vi "Convert_to_1D_Array.vi"(11 "Path":path) -> (3 "Array":string[](array[string]))   [LabVIEW 2017]
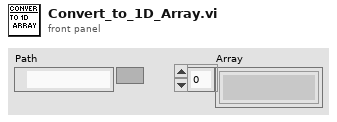
[diagram p1: front panel]
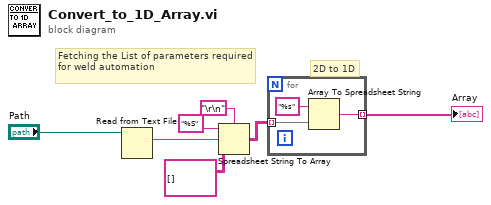
[diagram p0: block diagram]
diagram:
  # "2D to 1D"
  # "Fetching the List of parameters required for weld automation"
  n1 = Read from Text File(file (use dialog)="Path") -> (text=w2:string)  [unwired: 3 in, 3 out]
  n2 = Spreadsheet String To Array(delimiter (Tab)="\r\n", format string="%S", spreadsheet string=w2, array type (2D Dbl)=string[][] []) -> (array=w5:string[][])
  n3 = for {
    tunnel: w5 -> [w10] mode=indexing
    tunnel: [w8] -> w6 mode=indexing
    n4 = Array To Spreadsheet String(array=w10, 3:"%s" ("format string")) -> (spreadsheet string=w8:string)  [unwired: 1 in]
  }
  "Array" <- w6
